vi "Write Display Active Queue.vi"(10 "Display Active Queue":refnum<queue>, 11 "Assert Display in":refnum<class "Assert Display.lvclass">) -> (3 "Assert Display out":refnum<class "Assert Display.lvclass">)   [LabVIEW 2018, in "Assert API Components.lvlib" / "Assert Display.lvlib" / "Assert Display.lvclass"]
uses:
  Assert Display.lvclass
  Assert Display.lvclass/Assert Display.ctl
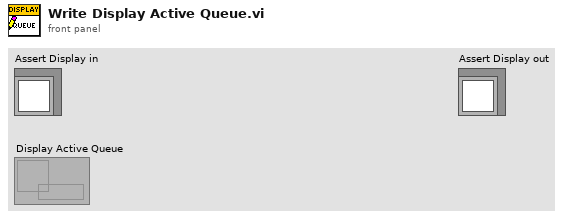
[diagram p1: front panel]
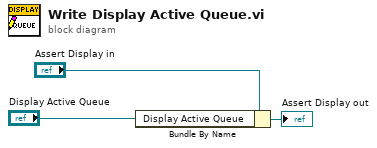
[diagram p0: block diagram]
diagram:
  n1 = Bundle By Name(cluster="Assert Display in", "Display Active Queue"="Display Active Queue") -> (→"Assert Display out":refnum<class "Assert Display.lvclass">)
